vi "old - R30-1-FPGA.vi"() -> ()   [LabVIEW 2016]
uses:
  <vilib>/LabVIEW Targets/FPGA/cRIO/shared/nicrio_ModuleControls/nicrio_cRIO-9871_BaudRateEnum.ctl
  <vilib>/LabVIEW Targets/FPGA/cRIO/shared/nicrio_ModuleControls/nicrio_cRIO-9871_ParityEnum.ctl
  <vilib>/LabVIEW Targets/FPGA/cRIO/shared/nicrio_ModuleControls/nicrio_cRIO-9871_StopBitsEnum.ctl
  <vilib>/LabVIEW Targets/FPGA/cRIO/shared/nicrio_ModuleControls/nicrio_cRIO-9871_DataBitsEnum.ctl
  <vilib>/Platform/TimedLoop/XDataNode/timing_clust.ctl
  <vilib>/Platform/TimedLoop/XDataNode/nitl_modes.ctl
  <vilib>/Platform/TimedLoop/XDataNode/wakeup.ctl
  <vilib>/rvi/FXPMathLib/basic elements/FxpIntAccumulator/subVIs/nifxpmath_IntAccumulator_SimConfig.ctl
  <vilib>/rvi/Emulation/niFpgaGetClockAttributes.vi
  <vilib>/rvi/Emulation/niFpgaSctlEmulationGetInTimedLoop.vi
  <vilib>/rvi/Emulation/niFpgaEmulationReportErrorSimple.vi
  <vilib>/rvi/eio/common/nirviEmuTemplateMethod_errors.vi
  <vilib>/rvi/Emulation/niFpgaCriticalErrorInLSC.vi
  <vilib>/rvi/Analysis/common/codeGenErrors/XNode/niFpgaXNodeCodeGenErrorHandle.vi
  <vilib>/rvi/FXPMathLib/basic elements/FxpIntAccumulator/simVIs/DllFxpIntAccumulator_sub.vi
  <vilib>/rvi/eio/common/nirviEmuTemplatePropertySet_noerrors.vi
  <vilib>/rvi/eio/common/nirviEmuTemplatePropertySet_errors.vi
  <vilib>/eio/EIONode/EIONode.xnode
  <vilib>/eio/EIOMethodNode/EIOMethodNode.xnode
  <vilib>/rvi/Analysis/measure/dc-rms/XNode/niFpgaDC-RMS.xnode
  <vilib>/Platform/TimedLoop/XDataNode/XDataNode.xnode
  <vilib>/rvi/FXPMathLib/basic elements/FxpIntAccumulator/XNode/nifxpmath_IntAccumulator.xnode
  <vilib>/rvi/FXPMathLib/FxpMul/XNode/nifxpmath_Multiplier.xnode
  <vilib>/eio/EIOPropertyNode/EIOPropertyNode.xnode
  <vilib>/Platform/TimedLoop/XDataNode/XDNodeRunTimeDep.lvlib
  <vilib>/rvi/FXPMathLib/sim/FxpSim.dll
  <vilib>/rvi/eio/common/nirviEmuTemplatePropertyGet_errors.vi
  <vilib>/rvi/eio/common/nirviEmuTemplatePropertyGet_noerrors.vi
panel:
  out "R30 Switch Image Convectron 1":u8[](array[numeric])
  out "R30 Switch Image Ion gauge 1":u8[](array[numeric])
  out "analog readback":fxp<+/-,26,5>[](array[numeric]) format="%.23g"
  out "Time since repurge":u8[](array[numeric])
  out "1st stage temp(k)":u8[](array[numeric])
  out "2nd stage":u8[](array[numeric])
  out "Time since pump on":u8[](array[numeric])
  out "Pump On":u8[](array[numeric])
  out "R30 Detector Convectron  1":u8[](array[numeric])
  out "R30 Detector Ion gauge 1":u8[](array[numeric])
  out "R30 ESA Convectron  1":u8[](array[numeric])
  out "R30 ESA Ion gauge 1":u8[](array[numeric])
  in  "y steerer magnet":fxp<+/-,20,5> format="%.17g"
  in  "analog output":fxp<+/-,64,32>[](array[numeric])=[0.0, 0.0, 0.0, 0.0, 0.0, 0.0, 0.0]
  out "Switch Ap IN":bool
  out "Switch Ap OUT2":bool
  out "Det Ap OUT":bool
  out "Det Ap IN":bool
  out "Detector  FC IN":bool
  out "Detector FC OUT":bool
  out "Switch magnet FC OUT":bool
  out "Switch magnet FC IN":bool
  in  "Switch magnet ap":bool
  in  "Detector AP":bool
  in  "Detector FC":bool
  in  "Switch magnet FC":bool
  out "Timed Out":bool
  out "Switch object tesla meter":u8[](array[numeric])
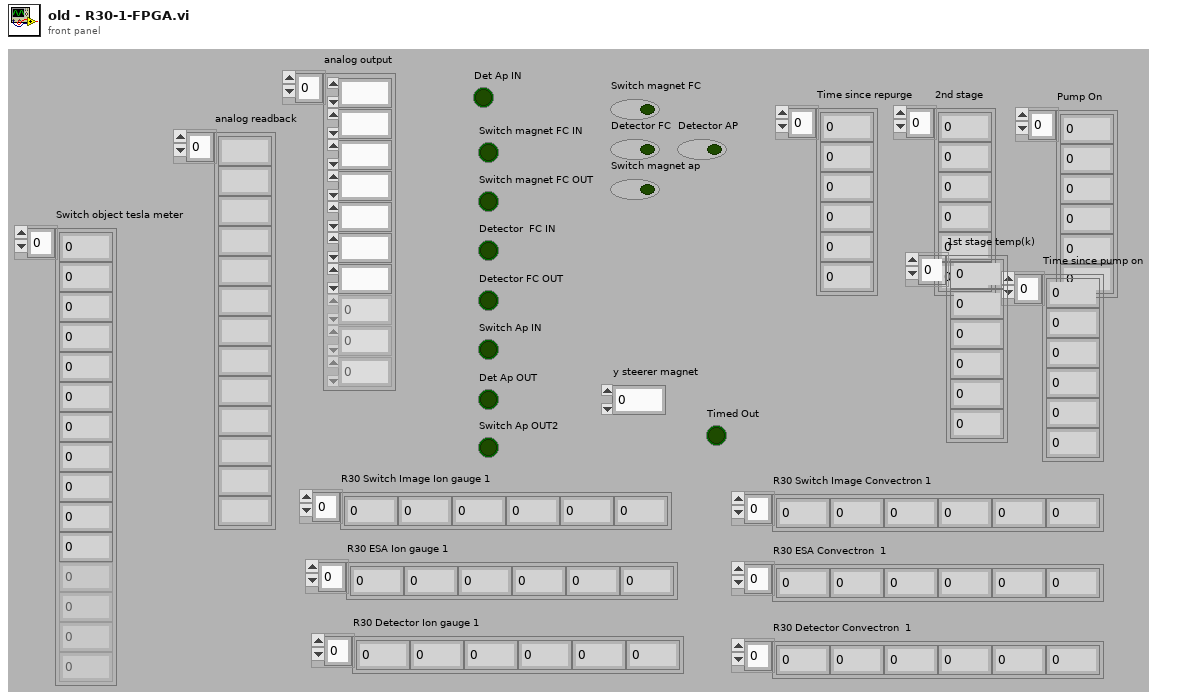
[diagram p1: front panel]
types:
  T1 = typedef "nicrio_cRIO-9871_StopBitsEnum.ctl" = enum8{"1", "1.5", "2"}
  T2 = typedef "nicrio_cRIO-9871_ParityEnum.ctl" = enum8{"None", "Odd", "Even", "Mark", "Space"}
  T3 = typedef "nicrio_cRIO-9871_DataBitsEnum.ctl" = enum8{"5", "6", "7", "8"}
  T4 = typedef "nicrio_cRIO-9871_BaudRateEnum.ctl" = enum16{"75 bps", "110 bps", "134 bps", "150 bps", "300 bps", "600 bps", "1200 bps", "1800 bps", "2400 bps", "4800 bps", "7200 bps", "9600 bps", "14.4 kbps", "19.2 kbps", "28.8 kbps", "38.4 kbps", "57.6 kbps", "115.2 kbps", "230.4 kbps", "460.8 kbps", "921.6 kbps"}
  T5 = typedef "XDNodeRunTimeDep.lvlib/timing_clust.ctl" = cluster{"Expected End [f-1]":u64, "Actual End [f-1]":u64, "Finished Late? [f-1]":bool, "Expected End [i-1]":u64, "Actual End [i-1]":u64, "Finished Late? [i-1]":bool, "Expected Start [i]":u64, "Actual Start [i]":u64, "Expected Start [f]":u64, "Actual Start [f]":u64, "Source Name":string, "Structure Name":string, "Period":i64, "Deadline":i64, "Offset":i64, "Start":i64, "Priority":i32, "Timeout":i32, "Mode":T6, "Wakeup Reason":T7, "Error":errorcluster, "Source Type":string, "Secondary Source Type":string, "Global End Time":u64, "Global Start Time":u64, "Frame Duration":u64, "Iteration Duration":u64, "Assigned CPU":i32, "I/O Scan Engine Mode":u32}
  T6 = typedef "XDNodeRunTimeDep.lvlib/nitl_modes.ctl" = enum32{"No Change", "Process missed periods, maintain original phase", "Discard missed periods, maintain original phase", "Process missed periods, ignore original phase", "Discard missed periods, ignore original phase"}
  T7 = typedef "XDNodeRunTimeDep.lvlib/wakeup.ctl" = enum32{"Normal", "Aborted", "Asynchronous wakeup", "Timing source error", "Timed loop error", "Timeout"}
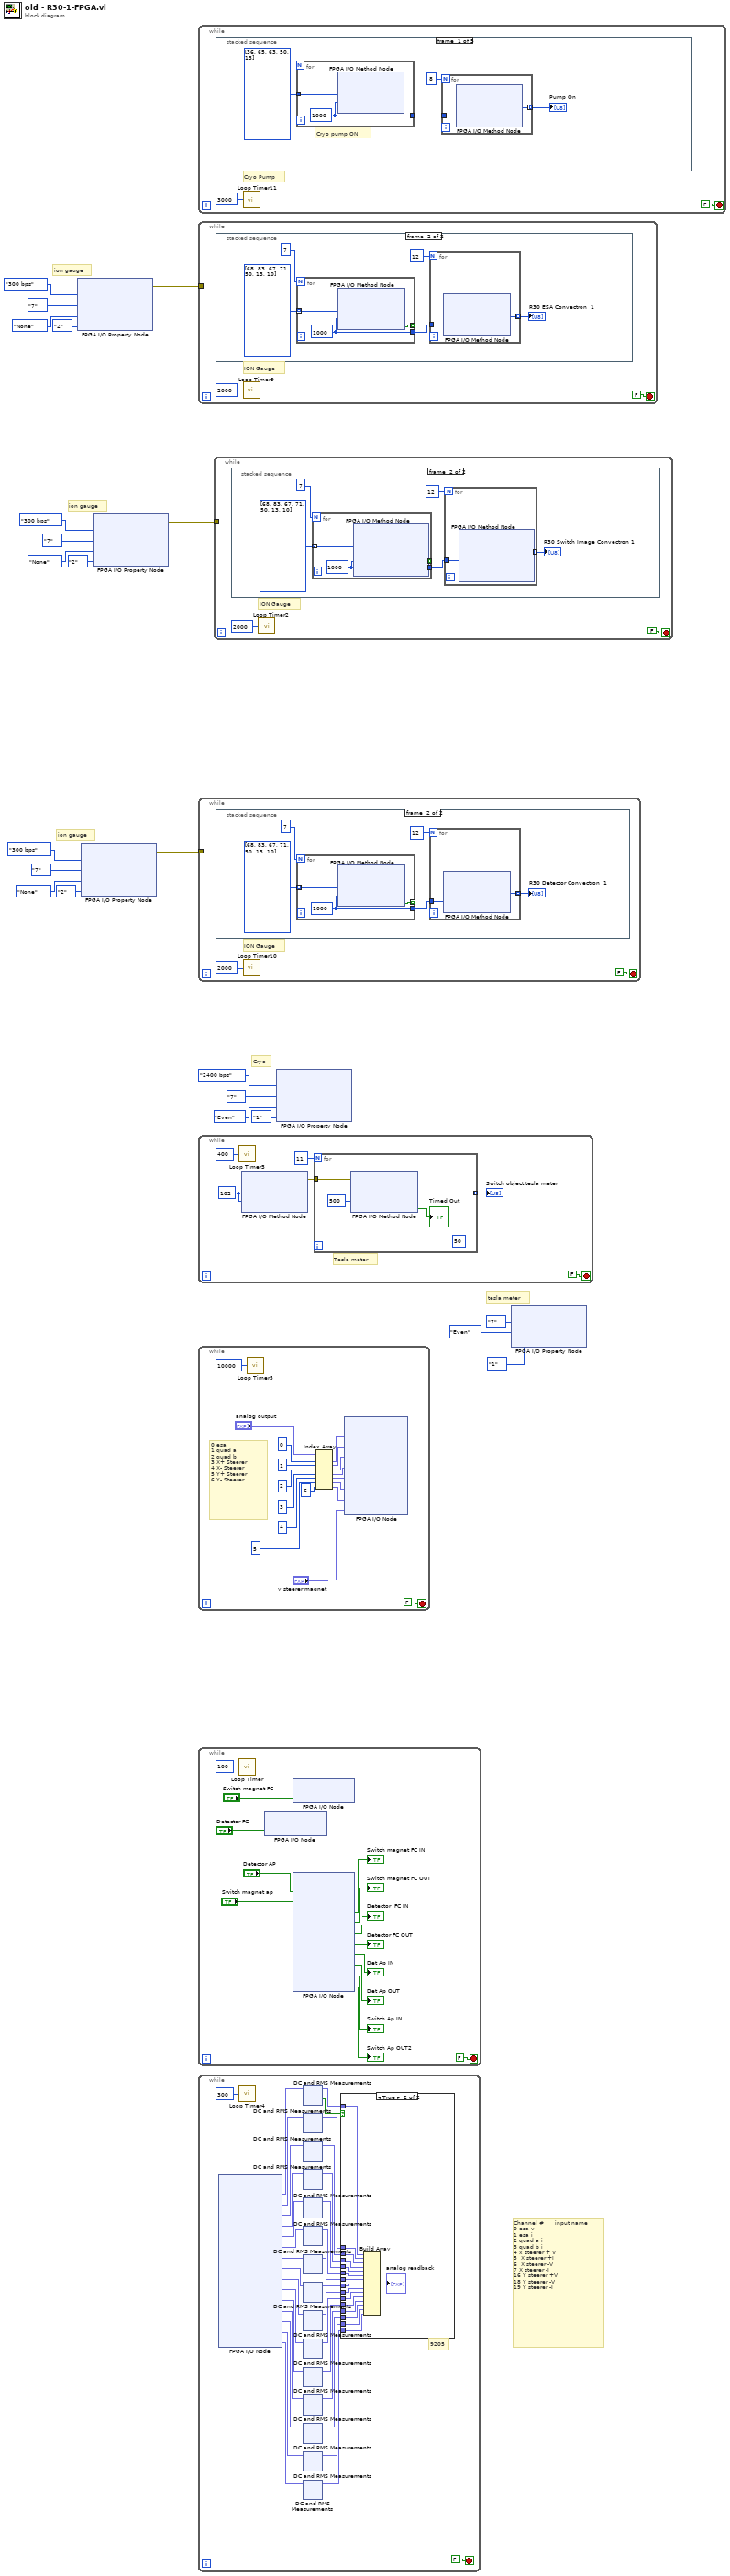
[diagram p0: block diagram]
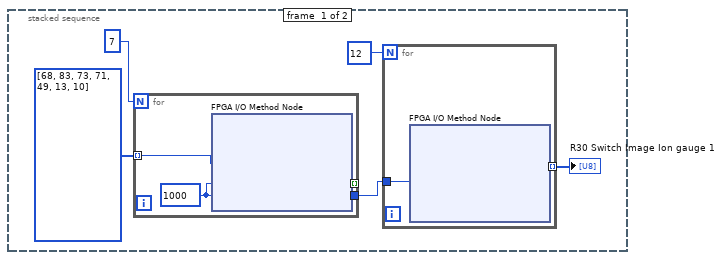
[diagram p2: hidden frame]
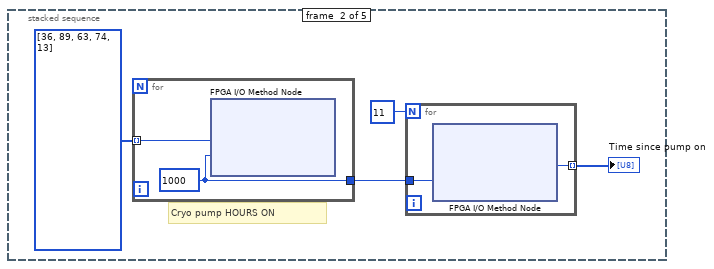
[diagram p3: hidden frame]
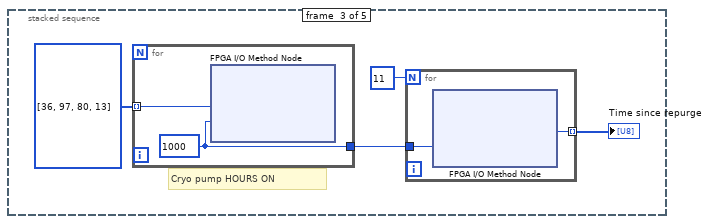
[diagram p4: hidden frame]
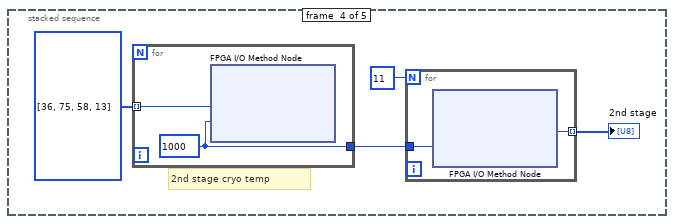
[diagram p5: hidden frame]
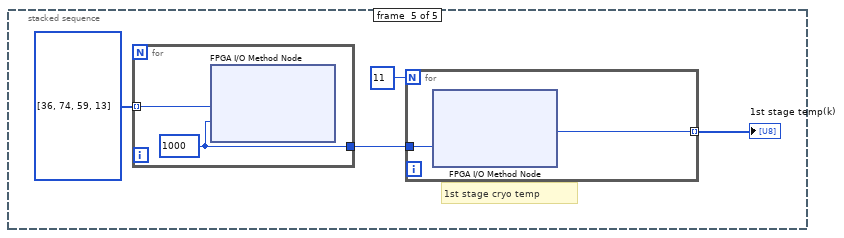
[diagram p6: hidden frame]
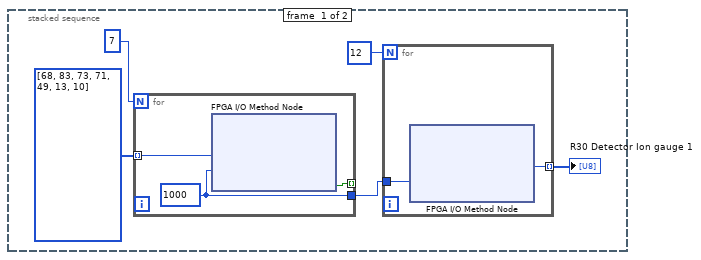
[diagram p7: hidden frame]
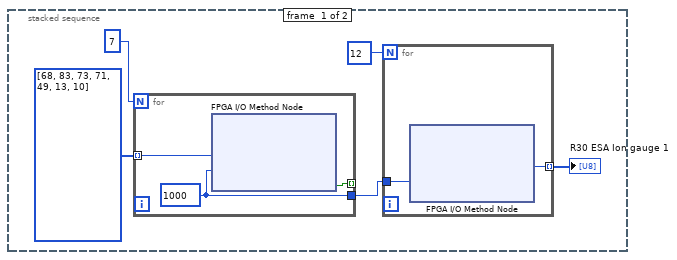
[diagram p8: hidden frame]
diagram:
  # "ion gauge"
  # "Channel #      input name\n0 esa v\n1 esa i\n2 quad a i\n3 quad b i\n4 x steerer + V\n5  X steerer +I\n6  X steerer -V\n7 X steerer -I\n16 Y steerer +V\n18 Y steerer -V\n19 Y steerer -I"
  # "tesla meter"
  # "Cryo"
  # "ion gauge"
  # "ion gauge"
  n1 = xnode "FPGA I/O Property Node"("Baud Rate"=nicrio_cRIO-9871_BaudRateEnum."300 bps", "Data Bits"=nicrio_cRIO-9871_DataBitsEnum."7", "Parity"=nicrio_cRIO-9871_ParityEnum."None", "Stop Bits"=nicrio_cRIO-9871_StopBitsEnum."2") -> ("error out"=w6:errorcluster)  [unwired: 2 in, 1 out]
  n2 = xnode "FPGA I/O Property Node"("Baud Rate"=nicrio_cRIO-9871_BaudRateEnum."300 bps", "Data Bits"=nicrio_cRIO-9871_DataBitsEnum."7", "Parity"=nicrio_cRIO-9871_ParityEnum."None", "Stop Bits"=nicrio_cRIO-9871_StopBitsEnum."2") -> ("error out"=w7:errorcluster)  [unwired: 2 in, 1 out]
  n3 = xnode "FPGA I/O Property Node"("Baud Rate"=nicrio_cRIO-9871_BaudRateEnum."300 bps", "Data Bits"=nicrio_cRIO-9871_DataBitsEnum."7", "Parity"=nicrio_cRIO-9871_ParityEnum."None", "Stop Bits"=nicrio_cRIO-9871_StopBitsEnum."2") -> ("error out"=w1:errorcluster)  [unwired: 2 in, 1 out]
  n4 = while {
    stop <- FALSE stop-if-true
    # "Cryo Pump"
    n5 = stacked-sequence {
      frame #0 {
        # "Cryo pump ON"
        n6 = for {
          tunnel: [w32] -> w28
          tunnel: u8[] [36, 65, 63, 50, 13] ("unsigned byte array") -> [w31] mode=indexing
          w32 = 1000 ("Timeout (ms)")
          n7 = xnode "FPGA I/O Method Node"("Data"=w31, "Timeout (ms)"=w32) -> ()  [unwired: 1 in, 2 out]
        }
        n8 = for {
          N: 8 -> [_]
          tunnel: w28 -> [w30]
          tunnel: [w29] -> w25 mode=indexing
          n9 = xnode "FPGA I/O Method Node"("Timeout (ms)"=w30) -> ("Data"=w29:u8)  [unwired: 1 in, 2 out]
        }
        "Pump On" <- w25
      }
      frame #1 {
        # "Cryo pump HOURS ON"
        n10 = for {
          tunnel: [w40] -> w36
          tunnel: u8[] [36, 89, 63, 74, 13] ("unsigned byte array") -> [w39] mode=indexing
          w40 = 1000 ("Timeout (ms)")
          n11 = xnode "FPGA I/O Method Node"("Data"=w39, "Timeout (ms)"=w40) -> ()  [unwired: 1 in, 2 out]
        }
        n12 = for {
          N: 11 -> [_]
          tunnel: w36 -> [w38]
          tunnel: [w37] -> w33 mode=indexing
          n13 = xnode "FPGA I/O Method Node"("Timeout (ms)"=w38) -> ("Data"=w37:u8)  [unwired: 1 in, 2 out]
        }
        "Time since pump on" <- w33
      }
      frame #2 {
        # "Cryo pump HOURS ON"
        n14 = for {
          tunnel: [w48] -> w44
          tunnel: u8[] [36, 97, 80, 13] ("unsigned byte array") -> [w47] mode=indexing
          w48 = 1000 ("Timeout (ms)")
          n15 = xnode "FPGA I/O Method Node"("Data"=w47, "Timeout (ms)"=w48) -> ()  [unwired: 1 in, 2 out]
        }
        n16 = for {
          N: 11 -> [_]
          tunnel: w44 -> [w46]
          tunnel: [w45] -> w41 mode=indexing
          n17 = xnode "FPGA I/O Method Node"("Timeout (ms)"=w46) -> ("Data"=w45:u8)  [unwired: 1 in, 2 out]
        }
        "Time since repurge" <- w41
      }
      frame #3 {
        # "2nd stage cryo temp"
        n18 = for {
          tunnel: [w56] -> w52
          tunnel: u8[] [36, 75, 58, 13] ("unsigned byte array") -> [w55] mode=indexing
          w56 = 1000 ("Timeout (ms)")
          n19 = xnode "FPGA I/O Method Node"("Data"=w55, "Timeout (ms)"=w56) -> ()  [unwired: 1 in, 2 out]
        }
        n20 = for {
          N: 11 -> [_]
          tunnel: w52 -> [w54]
          tunnel: [w53] -> w49 mode=indexing
          n21 = xnode "FPGA I/O Method Node"("Timeout (ms)"=w54) -> ("Data"=w53:u8)  [unwired: 1 in, 2 out]
        }
        "2nd stage" <- w49
      }
      frame #4 {
        # "1st stage cryo temp"
        n22 = for {
          tunnel: [w64] -> w60
          tunnel: u8[] [36, 74, 59, 13] ("unsigned byte array") -> [w63] mode=indexing
          w64 = 1000 ("Timeout (ms)")
          n23 = xnode "FPGA I/O Method Node"("Data"=w63, "Timeout (ms)"=w64) -> ()  [unwired: 1 in, 2 out]
        }
        n24 = for {
          N: 11 -> [_]
          tunnel: w60 -> [w62]
          tunnel: [w61] -> w57 mode=indexing
          n25 = xnode "FPGA I/O Method Node"("Timeout (ms)"=w62) -> ("Data"=w61:u8)  [unwired: 1 in, 2 out]
        }
        "1st stage temp(k)" <- w57
      }
    }
    n26 = call "Loop Timer11"("Count(mSec)"=u32 3000 ("Count(Ticks)")) -> ()  [unwired: 1 out]
  }
  n27 = while {
    tunnel: w6 -> [_]
    stop <- FALSE stop-if-true
    # "ION Gauge"
    n28 = stacked-sequence {
      frame #0 {
        n29 = for {
          N: 7 -> [_]
          tunnel: [w76] -> w71
          tunnel: [w75] -> _ mode=indexing
          tunnel: u8[] [68, 83, 73, 71, 49, 13, 10] ("unsigned byte array") -> [w74] mode=indexing
          w76 = 1000 ("Timeout (ms)")
          n30 = xnode "FPGA I/O Method Node"("Data"=w74, "Timeout (ms)"=w76) -> ("Timed Out"=w75:bool)  [unwired: 1 in, 1 out]
        }
        n31 = for {
          N: 12 -> [_]
          tunnel: w71 -> [w73]
          tunnel: [w72] -> w67 mode=indexing
          n32 = xnode "FPGA I/O Method Node"("Timeout (ms)"=w73) -> ("Data"=w72:u8)  [unwired: 1 in, 2 out]
        }
        "R30 ESA Ion gauge 1" <- w67
      }
      frame #1 {
        n33 = for {
          N: 7 -> [_]
          tunnel: [w86] -> w81
          tunnel: [w85] -> _ mode=indexing
          tunnel: u8[] [68, 83, 67, 71, 50, 13, 10] ("unsigned byte array") -> [w84] mode=indexing
          w86 = 1000 ("Timeout (ms)")
          n34 = xnode "FPGA I/O Method Node"("Data"=w84, "Timeout (ms)"=w86) -> ("Timed Out"=w85:bool)  [unwired: 1 in, 1 out]
        }
        n35 = for {
          N: 12 -> [_]
          tunnel: w81 -> [w83]
          tunnel: [w82] -> w77 mode=indexing
          n36 = xnode "FPGA I/O Method Node"("Timeout (ms)"=w83) -> ("Data"=w82:u8)  [unwired: 1 in, 2 out]
        }
        "R30 ESA Convectron  1" <- w77
      }
    }
    n37 = call "Loop Timer9"("Count(mSec)"=u32 2000 ("Count(Ticks)")) -> ()  [unwired: 1 out]
  }
  n38 = while {
    tunnel: w7 -> [_]
    stop <- FALSE stop-if-true
    # "ION Gauge"
    n39 = stacked-sequence {
      frame #0 {
        n40 = for {
          N: 7 -> [_]
          tunnel: [w98] -> w93
          tunnel: [w97] -> _ mode=indexing
          tunnel: u8[] [68, 83, 73, 71, 49, 13, 10] ("unsigned byte array") -> [w96] mode=indexing
          w98 = 1000 ("Timeout (ms)")
          n41 = xnode "FPGA I/O Method Node"("Data"=w96, "Timeout (ms)"=w98) -> ("Timed Out"=w97:bool)  [unwired: 1 in, 1 out]
        }
        n42 = for {
          N: 12 -> [_]
          tunnel: w93 -> [w95]
          tunnel: [w94] -> w89 mode=indexing
          n43 = xnode "FPGA I/O Method Node"("Timeout (ms)"=w95) -> ("Data"=w94:u8)  [unwired: 1 in, 2 out]
        }
        "R30 Detector Ion gauge 1" <- w89
      }
      frame #1 {
        n44 = for {
          N: 7 -> [_]
          tunnel: [w108] -> w103
          tunnel: [w107] -> _ mode=indexing
          tunnel: u8[] [68, 83, 67, 71, 50, 13, 10] ("unsigned byte array") -> [w106] mode=indexing
          w108 = 1000 ("Timeout (ms)")
          n45 = xnode "FPGA I/O Method Node"("Data"=w106, "Timeout (ms)"=w108) -> ("Timed Out"=w107:bool)  [unwired: 1 in, 1 out]
        }
        n46 = for {
          N: 12 -> [_]
          tunnel: w103 -> [w105]
          tunnel: [w104] -> w99 mode=indexing
          n47 = xnode "FPGA I/O Method Node"("Timeout (ms)"=w105) -> ("Data"=w104:u8)  [unwired: 1 in, 2 out]
        }
        "R30 Detector Convectron  1" <- w99
      }
    }
    n48 = call "Loop Timer10"("Count(mSec)"=u32 2000 ("Count(Ticks)")) -> ()  [unwired: 1 out]
  }
  n49 = while {
    stop <- FALSE stop-if-true
    w111 = u8 102 ("Data")
    # "Tesla meter"
    n50 = call "Loop Timer3"("Count(mSec)"=u32 400) -> ()  [unwired: 1 out]
    n51 = xnode "FPGA I/O Method Node"("Data"=w111, "Timeout (ms)"=w111) -> ("error out"=w110:errorcluster)  [unwired: 2 in, 2 out]
    n52 = for {
      N: 11 ("Numeric 3") -> [_]
      tunnel: [w116] -> w112 mode=indexing
      tunnel: w110 -> [w115]
      (unwired) 50 ("Timeout")
      n53 = xnode "FPGA I/O Method Node"("error in"=w115, "Timeout (ms)"=500) -> ("Data"=w116:u8, "Timed Out"=→"Timed Out":bool)  [unwired: 1 in, 2 out]
    }
    "Switch object tesla meter" <- w112
  }
  n54 = while {
    stop <- FALSE stop-if-true
    # "0 esa\n1 quad a\n2 quad b\n3 X+ Steerer\n4 X- Steerer\n5 Y+ Steerer\n6 Y- Steerer"
    n55 = call "Loop Timer5"("Count(Ticks)"=u32 10000 ("Count(mSec)")) -> ()  [unwired: 1 out]
    n56 = Index Array(array="analog output", index #1=0 ("index"), index #2=1 ("index"), index #3=2 ("index"), index #4=3 ("index"), index #5=4 ("index"), index #6=5 ("index"), index #7=6 ("index")) -> (element #1=w126:fxp<+/-,64,32>, element #2=w125:fxp<+/-,64,32>, element #3=w124:fxp<+/-,64,32>, element #4=w123:fxp<+/-,64,32>, element #5=w122:fxp<+/-,64,32>, element #6=w121:fxp<+/-,64,32>, element #7=w120:fxp<+/-,64,32>)
    n57 = xnode "FPGA I/O Node"("Mod1/AO0"=w126, "Mod1/AO1"=w125, "Mod1/AO2"=w124, "Mod1/AO3"=w123, "Mod1/AO4"=w122, "Mod1/AO5"=w121, "Mod1/AO6"=w120, "Mod1/AO7"="y steerer magnet") -> ()  [unwired: 8 in, 8 out]
  }
  n58 = while {
    stop <- FALSE stop-if-true
    n59 = call "Loop Timer"("Count(mSec)"=u32 100 ("Count(uSec)")) -> ()  [unwired: 1 out]
    n60 = xnode "FPGA I/O Node"("Mod8/CH1"="Detector FC") -> ()  [unwired: 1 in, 1 out]
    n61 = xnode "FPGA I/O Node"("Mod8/CH0"="Switch magnet FC") -> ()  [unwired: 1 in, 1 out]
    n62 = xnode "FPGA I/O Node"("Mod8/CH2"="Detector AP", "Mod8/CH3"="Switch magnet ap") -> ("Mod7/DI0"=→"Switch magnet FC IN":bool, "Mod7/DI1"=→"Switch magnet FC OUT":bool, "Mod7/DI2"=→"Detector  FC IN":bool, "Mod7/DI3"=→"Detector FC OUT":bool, "Mod7/DI4"=→"Det Ap IN":bool, "Mod7/DI5"=→"Det Ap OUT":bool, "Mod7/DI6"=→"Switch Ap IN":bool, "Mod7/DI7"=→"Switch Ap OUT2":bool)  [unwired: 10 in, 10 out]
  }
  n63 = while {
    stop <- FALSE stop-if-true
    # "9205"
    n64 = xnode "FPGA I/O Node"() -> ("Mod2/AI0"=w180:fxp<+/-,26,5>, "Mod2/AI1"=w178:fxp<+/-,26,5>, "Mod2/AI2"=w176:fxp<+/-,26,5>, "Mod2/AI3"=w174:fxp<+/-,26,5>, "Mod2/AI4"=w172:fxp<+/-,26,5>, "Mod2/AI5"=w170:fxp<+/-,26,5>, "Mod2/AI6"=w168:fxp<+/-,26,5>, "Mod2/AI7"=w166:fxp<+/-,26,5>, "Mod2/AI16"=w164:fxp<+/-,26,5>, "Mod2/AI17"=w162:fxp<+/-,26,5>, "Mod2/AI18"=w160:fxp<+/-,26,5>, "Mod2/AI19"=w158:fxp<+/-,26,5>, "Mod2/AI20"=w156:fxp<+/-,26,5>, "Mod2/AI21"=w154:fxp<+/-,26,5>, "Mod2/AI22"=w152:fxp<+/-,26,5>)  [unwired: 15 in, 15 out]
    n65 = call "Loop Timer4"("Count(Ticks)"=u32 300) -> ()  [unwired: 1 out]
    n66 = xnode "DC and RMS Measurements"("input data"=w180) -> ("DC"=w179:fxp<+/-,26,5>, "output valid"=w181:bool)  [unwired: 1 in]
    n67 = xnode "DC and RMS Measurements"("input data"=w178) -> ("DC"=w177:fxp<+/-,26,5>)  [unwired: 1 in, 1 out]
    n68 = xnode "DC and RMS Measurements"("input data"=w176) -> ("DC"=w175:fxp<+/-,26,5>)  [unwired: 1 in, 1 out]
    n69 = xnode "DC and RMS Measurements"("input data"=w174) -> ("DC"=w173:fxp<+/-,26,5>)  [unwired: 1 in, 1 out]
    n70 = xnode "DC and RMS Measurements"("input data"=w172) -> ("DC"=w171:fxp<+/-,26,5>)  [unwired: 1 in, 1 out]
    n71 = xnode "DC and RMS Measurements"("input data"=w170) -> ("DC"=w169:fxp<+/-,26,5>)  [unwired: 1 in, 1 out]
    n72 = xnode "DC and RMS Measurements"("input data"=w168) -> ("DC"=w167:fxp<+/-,26,5>)  [unwired: 1 in, 1 out]
    n73 = xnode "DC and RMS Measurements"("input data"=w166) -> ("DC"=w165:fxp<+/-,26,5>)  [unwired: 1 in, 1 out]
    n74 = xnode "DC and RMS Measurements"("input data"=w164) -> ("DC"=w163:fxp<+/-,26,5>)  [unwired: 1 in, 1 out]
    n75 = xnode "DC and RMS Measurements"("input data"=w162) -> ("DC"=w161:fxp<+/-,26,5>)  [unwired: 1 in, 1 out]
    n76 = xnode "DC and RMS Measurements"("input data"=w160) -> ("DC"=w159:fxp<+/-,26,5>)  [unwired: 1 in, 1 out]
    n77 = xnode "DC and RMS Measurements"("input data"=w158) -> ("DC"=w157:fxp<+/-,26,5>)  [unwired: 1 in, 1 out]
    n78 = xnode "DC and RMS Measurements"("input data"=w156) -> ("DC"=w155:fxp<+/-,26,5>)  [unwired: 1 in, 1 out]
    n79 = xnode "DC and RMS Measurements"("input data"=w154) -> ("DC"=w153:fxp<+/-,26,5>)  [unwired: 1 in, 1 out]
    n80 = xnode "DC and RMS Measurements"("input data"=w152) -> ("DC"=w151:fxp<+/-,26,5>)  [unwired: 1 in, 1 out]
    n81 = case shown="True" w181 {
      tunnel: w179 -> [_ w358]
      tunnel: w177 -> [_ w357]
      tunnel: w175 -> [_ w356]
      tunnel: w173 -> [_ w355]
      tunnel: w171 -> [_ w354]
      tunnel: w169 -> [_ w353]
      tunnel: w167 -> [_ w352]
      tunnel: w165 -> [_ w351]
      tunnel: w163 -> [_ w350]
      tunnel: w161 -> [_ w349]
      tunnel: w159 -> [_ w348]
      tunnel: w157 -> [_ w347]
      tunnel: w155 -> [_ w346]
      tunnel: w153 -> [_ w345]
      tunnel: w151 -> [_ w344]
      frame False {
      }
      frame True {
        n82 = Build Array(w358, w357, w356, w355, w354, w353, w352, w351, w350, w349, w348, w347, w346, w345, w344) -> (→"analog readback":fxp<+/-,26,5>[])
      }
    }
  }
  n83 = while {
    tunnel: w1 -> [_]
    stop <- FALSE stop-if-true
    # "ION Gauge"
    n84 = stacked-sequence {
      frame #0 {
        n85 = for {
          N: 7 -> [_]
          tunnel: [w1411] -> w1406
          tunnel: [w1410] -> _ mode=indexing
          tunnel: u8[] [68, 83, 73, 71, 49, 13, 10] ("unsigned byte array") -> [w1409] mode=indexing
          w1411 = 1000 ("Timeout (ms)")
          n86 = xnode "FPGA I/O Method Node"("Data"=w1409, "Timeout (ms)"=w1411) -> ("Timed Out"=w1410:bool)  [unwired: 1 in, 1 out]
        }
        n87 = for {
          N: 12 -> [_]
          tunnel: w1406 -> [w1408]
          tunnel: [w1407] -> w1402 mode=indexing
          n88 = xnode "FPGA I/O Method Node"("Timeout (ms)"=w1408) -> ("Data"=w1407:u8)  [unwired: 1 in, 2 out]
        }
        "R30 Switch Image Ion gauge 1" <- w1402
      }
      frame #1 {
        n89 = for {
          N: 7 -> [_]
          tunnel: [w1421] -> w1416
          tunnel: [w1420] -> _ mode=indexing
          tunnel: u8[] [68, 83, 67, 71, 50, 13, 10] ("unsigned byte array") -> [w1419] mode=indexing
          w1421 = 1000 ("Timeout (ms)")
          n90 = xnode "FPGA I/O Method Node"("Data"=w1419, "Timeout (ms)"=w1421) -> ("Timed Out"=w1420:bool)  [unwired: 1 in, 1 out]
        }
        n91 = for {
          N: 12 -> [_]
          tunnel: w1416 -> [w1418]
          tunnel: [w1417] -> w1412 mode=indexing
          n92 = xnode "FPGA I/O Method Node"("Timeout (ms)"=w1418) -> ("Data"=w1417:u8)  [unwired: 1 in, 2 out]
        }
        "R30 Switch Image Convectron 1" <- w1412
      }
    }
    n93 = call "Loop Timer2"("Count(mSec)"=u32 2000 ("Count(Ticks)")) -> ()  [unwired: 1 out]
  }
  n94 = xnode "FPGA I/O Property Node"("Baud Rate"=nicrio_cRIO-9871_BaudRateEnum."2400 bps", "Data Bits"=nicrio_cRIO-9871_DataBitsEnum."7", "Parity"=nicrio_cRIO-9871_ParityEnum."Even", "Stop Bits"=nicrio_cRIO-9871_StopBitsEnum."1") -> ()  [unwired: 1 in, 1 out]
  n95 = xnode "FPGA I/O Property Node"("Data Bits"=nicrio_cRIO-9871_DataBitsEnum."7", "Parity"=nicrio_cRIO-9871_ParityEnum."Even", "Stop Bits"=nicrio_cRIO-9871_StopBitsEnum."1") -> ()  [unwired: 1 in, 1 out]
